vi "error_check_magnetoresistance.vi"(8 "States in":T1, 11 "Boolean":bool) -> (3 "States out":T1)   [LabVIEW 2017]
uses:
  controls/State.ctl
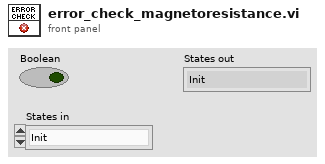
[diagram p1: front panel]
types:
  T1 = typedef "State.ctl" = enum16{"Init", "Idle", "Starting meas", "Running", "Stopping meas", "Shutdown"}
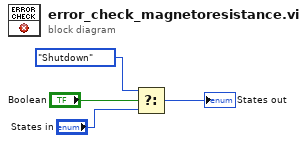
[diagram p0: block diagram]
diagram:
  n1 = Select(t=State."Shutdown", s="Boolean", f="States in") -> (s? t:f=→"States out":T1)
